vi "USBData_terminate.vi"(8 "error in (no error)":errorcluster, 11 "USBData in":refnum<class "USBData.lvclass">) -> (0 "error out":errorcluster, 3 "USBData out":refnum<class "USBData.lvclass">)   [LabVIEW 2017, in "USBData.lvclass"]
uses:
  USBData.lvclass
  USBData.lvclass/USBData.ctl
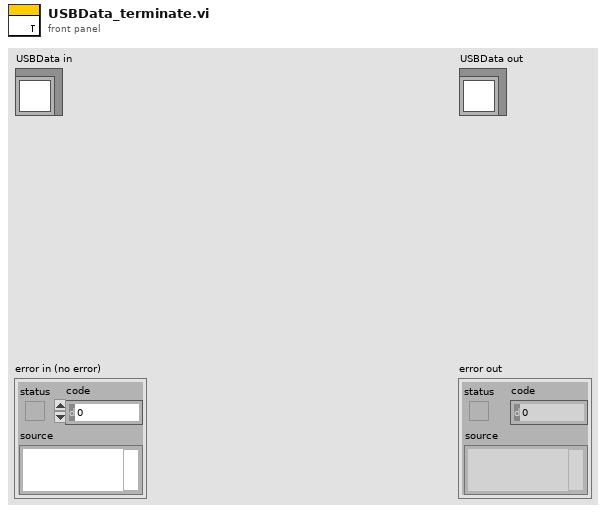
[diagram p1: front panel]
types:
  T1 = enum16{"Intialized", "Waiting", "Measuring", "Terminated"}
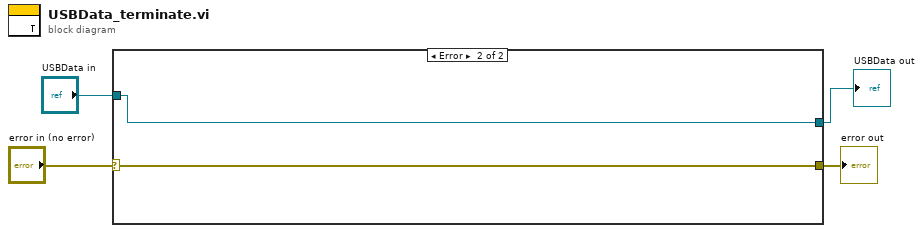
[diagram p0: block diagram]
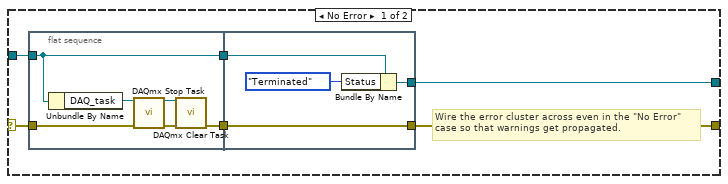
[diagram p2: hidden frame]
diagram:
  n1 = case shown="Error" "error in (no error)" {
    selector: "error in (no error)" -> [w10 w22]
    tunnel: [w9 w22] -> w3
    tunnel: "USBData in" -> [w8 w21]
    tunnel: [w6 w21] -> w1
    frame No Error {
      # "Wire the error cluster across even in the \"No Error\"\ncase so that warnings get propagated."
      n2 = flat-sequence {
        tunnel: w10 -> [w15]
        tunnel: w8 -> [w11]
        tunnel: [w12] -> w7
        tunnel: [w11] -> w5
        tunnel: [w20] -> w9
        tunnel: w7 -> [w20]
        tunnel: [w18] -> w6
        tunnel: w5 -> [w17]
        frame #0 {
          n3 = Unbundle By Name(w11) -> ("DAQ_task"=w16:refnum<k21>)
          n4 = call "DAQmx Stop Task.vi"("task/channels in"=w16, "error in"=w15) -> ("task out"=w13:refnum<k21>, "error out"=w14:errorcluster)  [unwired: 12 in]
          n5 = call "DAQmx Clear Task.vi"("task in"=w13, "error in"=w14) -> ("error out"=w12:errorcluster)  [unwired: 13 in]
        }
        frame #1 {
          n6 = Bundle By Name(cluster=w17, "Status"=T1."Terminated") -> (w18:refnum<class "USBData.lvclass">)
        }
      }
    }
    frame Error {
    }
  }
  "error out" <- w3
  "USBData out" <- w1
